vi "Get Engine Simulation Toolkit Custom Device.vi"(8 "error in (no error)":errorcluster, 11 "EST Custom Device in":refnum<k24>) -> (0 "error out":errorcluster, 2 "Settings":T1 {"Rate decimation" min=1}, 3 "EST Custom Device out":refnum<k24>)   [LabVIEW 2015, in "Engine Simulation Toolkit Scripting API.lvlib"]
uses:
  Engine Simulation Toolkit Scripting API.lvlib
  Engine Simulation Toolkit Custom Device Settings.ctl
  NationalInstruments.VeriStand.SystemDefinitionAPI
  Shared/Properties.vi
  <vilib>/NI Veristand/Custom Device API/Get Item Property (I32).vi
  Shared/Engine Simulation Toolkit Shared.lvlib
  <vilib>/NI VeriStand/Custom Device API/Custom Device API.lvlib
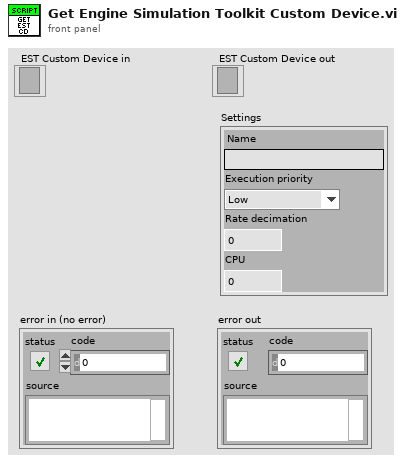
[diagram p1: front panel]
types:
  T1 = typedef "Engine Simulation Toolkit Scripting API.lvlib/Engine Simulation Toolkit Custom Device Settings.ctl" = cluster{"Name":string, "Execution priority":enum16{"Low", "Medium", "High"}, "Rate decimation":i32, "CPU":i32}
  T2 = typedef "Custom Device API.lvlib/Custom Device Item Info.ctl" = cluster{"Name":string, "Is Channel":bool, "GUID":string, "Is Waveform":bool}
  T3 = typedef "Custom Device API.lvlib/Custom Device Item Ref.ctl" = u64
  T4 = typedef "Custom Device API.lvlib/Custom Device Timed Loop Priority.ctl" = enum32{"Low", "Medium", "High"}
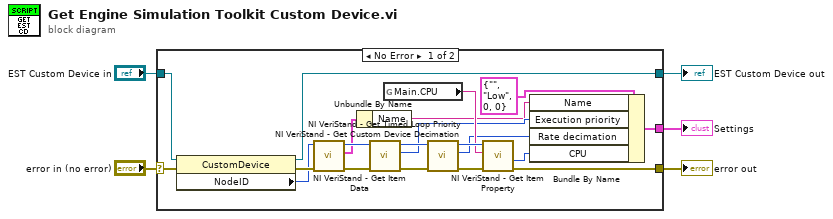
[diagram p0: block diagram]
diagram:
  n1 = case shown="No Error" "error in (no error)" {
    selector: "error in (no error)" -> [w18 w27]
    tunnel: [w25 w27] -> w5
    tunnel: [w19 w26] -> w4
    tunnel: "EST Custom Device in" -> [w17 w26]
    tunnel: [w16 _] -> w1
    frame No Error {
      n2 = property class="CustomDevice"(reference=w17, error in=w18) -> (reference out=w19:refnum<k24>, error out=w11:errorcluster, "NodeID"=w9:u64)
      n3 = call <vilib>:"NI VeriStand - Get Item Data.vi"("error in (no error)"=w11, "Item Ref in"=w9) -> ("error out"=w10:errorcluster, "Item Info"=w7:T2, "Item Ref out"=w8:T3)  [unwired: 6 in, 1 out]
      n4 = Unbundle By Name(w7) -> ("Name"=w6:string)
      n5 = call <vilib>:"NI VeriStand - Get Timed Loop Priority.vi"("error in (no error)"=w10, "Device Ref in"=w8) -> ("error out"=w24:errorcluster, "Priority"=w14:T4, "Device Ref out"=w20:T3)  [unwired: 7 in]
      n6 = global read "Properties.vi" "Main.CPU"() -> (w21:string)
      n7 = call <vilib>:"NI VeriStand - Get Custom Device Decimation.vi"("error in (no error)"=w24, "Device Ref in"=w20) -> ("error out"=w23:errorcluster, "Decimation"=w12:i32, "Device Ref out"=w22:T3)  [unwired: 7 in]
      n8 = call-poly <vilib>:"NI VeriStand - Get Item Property.vi"("error in (no error)"=w23, "Property Name"=w21, "Item Ref in"=w22) -> ("error out"=w25:errorcluster, "Value"=w13:i32)  [unwired: 5 in, 2 out]
      n9 = Bundle By Name(cluster=T1 {"Name"="", "Execution priority"=enum."Low", "Rate decimation"=0, "CPU"=0} ("Settings"), "Name"=w6, "Execution priority"=w14, "Rate decimation"=w12, "CPU"=w13) -> (w16:T1)
    }
    frame Error {
    }
  }
  "Settings" <- w1
  "error out" <- w5
  "EST Custom Device out" <- w4
